vi "ROI entry-Draw all ROI.vi"(8 "error in (no error)":errorcluster) -> (0 "error out":errorcluster)   [LabVIEW 2020]
uses:
  Typedefs/ROI management FG states.ctl
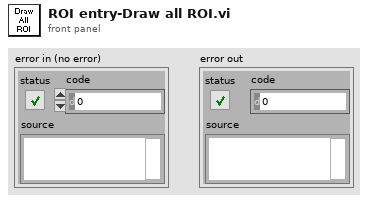
[diagram p1: front panel]
types:
  T1 = typedef "ROI management FG states.ctl" = enum16{"Read", "Write", "Write-from dataset", "Clear Last", "Clear All", "Delete ROI", "Update ROIs time", "Reload last ROI set", "Modify ROI Parameters", "Offset all ROI", "Offset visible ROI", "Modify Dwell Time", "Modify Laser Power"}
  T2 = typedef "IMAQ Image.ctl" = refnum<image>
  T3 = typedef "ROI parameters data type.ctl" = cluster{"ROI index":dbl, "ROI ID":dbl, "ROI Time (ns)":dbl, "Pixels in ROI":dbl, "X start":dbl, "Y start":dbl, "Z start":dbl, "X stop":dbl, "Y stop":dbl, "Z stop":dbl, "Angle (deg)":dbl, "Composite ID":dbl, "Number of lines":dbl, "Frame Size":dbl, "Zoom":dbl, "Laser Power (%)":dbl, "ROI group ID":dbl, "Resolution":dbl, "Dwell Time per pixel":dbl, "Pixels per miniscan":dbl, "Original FOV (um)":dbl, "Apparent Frame Size":dbl, "Z Plane Idx":i32[], "Z Plane codes":i32[]}
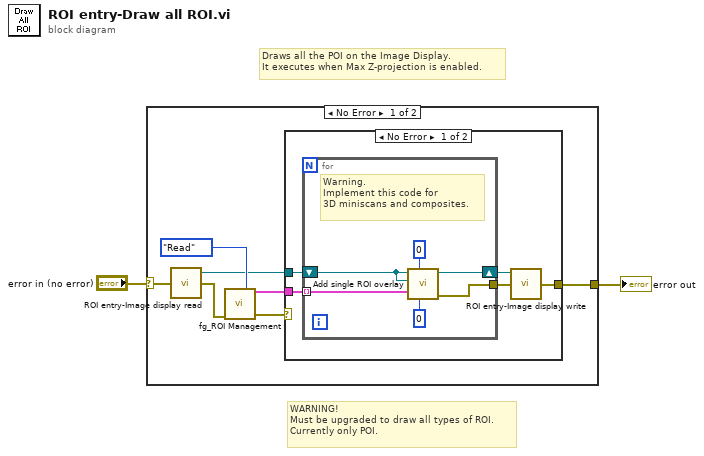
[diagram p0: block diagram]
diagram:
  # "WARNING!\nMust be upgraded to draw all types of ROI.\nCurrently only POI."
  # "Draws all the POI on the Image Display.\nIt executes when Max Z-projection is enabled."
  n1 = case shown="No Error" "error in (no error)" {
    selector: "error in (no error)" -> [w4 w22]
    tunnel: [w3 w22] -> w2
    frame No Error {
      n2 = call "ROI entry-Image display read.vi"("error in (no error)"=w4) -> ("error out"=w5:errorcluster, "CurrentImage"=w7:T2)  [unwired: 3 in]
      n3 = call "fg_ROI Management.vi"("Function"=ROI_management_FG_states."Read", "error in (no error)"=w5) -> ("ROI Setup"=w8:T3[], "error out"=w6:errorcluster)  [unwired: 7 in, 5 out]
      n4 = case shown="No Error" w6 {
        selector: w6 -> [_ w21]
        tunnel: w8 -> [w14 _]
        tunnel: w7 -> [w13 _]
        tunnel: [w11 w21] -> w3
        frame No Error {
          n5 = for {
            tunnel: w14 -> [w18] mode=indexing
            shift-right: [w16] -> w12
            shift-left: w13 -> [w17]
            tunnel: [w15] -> w10
            # "Warning.\nImplement this code for\n3D miniscans and composites."
            n6 = call "Add single ROI overlay.vi"("Abs. index of selected Z-plane (unity-based)"=0, "Number of Z-planes"=0, "ROI Properties"=w18, "Image2"=w17, "Image1"=w17) -> ("Error out"=w15:errorcluster, "Image1 Out"=w16:T2)  [unwired: 4 in, 1 out]
          }
          n7 = call "ROI entry-Image display write.vi"("error in (no error)"=w10, "Value"=w12) -> ("error out"=w11:errorcluster)  [unwired: 3 in]
        }
        frame Error {
        }
      }
    }
    frame Error {
    }
  }
  "error out" <- w2
